vi "Run All Custom Tests.vi"(7 "Main VI":path, 8 "Error In":errorcluster, 9 "Grader Result in":T6, 10 "Challenge Config":T5, 11 "VIChallenge Config":T1={"AWS Credentials"={"AWSAccessKeyId"="", "Secret Key"=""}, "AWS Account Number"="", "SQS Jobs"=refnum, "SQS Status"=refnum, "Source Dir"=path "", "Working Dir"=path "", "Output Dir"=path "", "Archive Dir"=path "", "job"={"job_id"="", "challenge_id"="", "user_id"="", "s3_source_bucket"="", "s3_source_directory"="", "s3_source_filename"="", "status_queue_name"="", "username"=""}, "Database Ref"=refnum, "Challenge Dir"=path "", "Challenges"=[]}) -> (0 "Error Out":errorcluster, 1 "Grader Result":T6, 2 "Challenge Config":T5, 3 "VIChallenge Config":T1)   [LabVIEW 2013, in "VIChallenge.lvlib"]
doc: "This VI runs all custom tests for the given challenge and returns a single result."
uses:
  <vilib>/LabVIEW Hacker/VIChallenge/VIChallenge.lvlib
  <vilib>/LabVIEW Hacker/VIChallenge/Private/Grader/Type Defs/Grader Result.ctl
  <vilib>/LabVIEW Hacker/VIChallenge/Private/Type Defs/Database/Score.ctl
  <vilib>/LabVIEW Hacker/VIChallenge/Private/Grader/Type Defs/UTF Status.ctl
  <vilib>/LabVIEW Hacker/VIChallenge/Private/Grader/Type Defs/Challenge.ctl
  <vilib>/LabVIEW Hacker/VIChallenge/Private/Type Defs/VIChallenge Config.ctl
  <vilib>/National Instruments/NI Amazon Web Services (AWS) Toolkit for LabVIEW/SQS/VI Source/AWS SQS Class/AWS_SQS.lvclass
  <vilib>/National Instruments/NI Amazon Web Services (AWS) Toolkit for LabVIEW/AWS Core Lib/VI Source/Canonicals/AWS_Core Canonical Credentials/Canonical Credentials.lvclass
  <vilib>/National Instruments/NI Amazon Web Services (AWS) Toolkit for LabVIEW/AWS Core Lib/VI Source/Canonicals/AWS_Core Canonical Required Parameters/Canonical Required Parameters.lvclass
  <vilib>/National Instruments/NI Amazon Web Services (AWS) Toolkit for LabVIEW/SQS/VI Source/Canonicals/Canonical CreateQueue/Canonical CreateQueue.lvclass
  <vilib>/National Instruments/NI Amazon Web Services (AWS) Toolkit for LabVIEW/SQS/VI Source/Canonicals/Canonical ListQueues/Canonical ListQueues.lvclass
  <vilib>/National Instruments/NI Amazon Web Services (AWS) Toolkit for LabVIEW/SQS/VI Source/Canonicals/Canonical AddPermission/Canonical AddPermission.lvclass
  <vilib>/National Instruments/NI Amazon Web Services (AWS) Toolkit for LabVIEW/SQS/VI Source/Canonicals/Canonical ChangeMessageVisibility/Canonical ChangeMessageVisibility.lvclass
  <vilib>/National Instruments/NI Amazon Web Services (AWS) Toolkit for LabVIEW/SQS/VI Source/Canonicals/Canonical ChangeMessageVisibilityBatch/Canonical ChangeMessageVisibilityBatch.lvclass
  <vilib>/National Instruments/NI Amazon Web Services (AWS) Toolkit for LabVIEW/SQS/VI Source/Canonicals/Canonical DeleteMessage/Canonical DeleteMessage.lvclass
  <vilib>/National Instruments/NI Amazon Web Services (AWS) Toolkit for LabVIEW/SQS/VI Source/Canonicals/Canonical DeleteMessageBatch/Canonical DeleteMessageBatch.lvclass
  <vilib>/National Instruments/NI Amazon Web Services (AWS) Toolkit for LabVIEW/SQS/VI Source/Canonicals/Canonical GetQueueAttributes/Canonical GetQueueAttributes.lvclass
  <vilib>/National Instruments/NI Amazon Web Services (AWS) Toolkit for LabVIEW/SQS/VI Source/Canonicals/Canonical GetQueueUrl/Canonical GetQueueUrl.lvclass
  <vilib>/National Instruments/NI Amazon Web Services (AWS) Toolkit for LabVIEW/SQS/VI Source/Canonicals/Canonical ReceiveMessage/Canonical ReceiveMessage.lvclass
  <vilib>/National Instruments/NI Amazon Web Services (AWS) Toolkit for LabVIEW/SQS/VI Source/Canonicals/Canonical RemovePermission/Canonical RemovePermission.lvclass
  <vilib>/National Instruments/NI Amazon Web Services (AWS) Toolkit for LabVIEW/SQS/VI Source/Canonicals/Canonical SendMessage/Canonical SendMessage.lvclass
  <vilib>/National Instruments/NI Amazon Web Services (AWS) Toolkit for LabVIEW/SQS/VI Source/Canonicals/Canonical SendMessageBatch/Canonical SendMessageBatch.lvclass
  <vilib>/National Instruments/NI Amazon Web Services (AWS) Toolkit for LabVIEW/SQS/VI Source/Canonicals/Canonical SetQueueAttributes/Canonical SetQueueAttributes.lvclass
  <vilib>/National Instruments/NI Amazon Web Services (AWS) Toolkit for LabVIEW/AWS Core Lib/VI Source/Typedefs/AWS_AWS Credentials.ctl
  <vilib>/LabVIEW Hacker/VIChallenge/Private/Type Defs/JSON_job.ctl
  <vilib>/addons/database/Connection.llb/Conn ObjectReference.ctl
  <vilib>/National Instruments/NI Amazon Web Services (AWS) Toolkit for LabVIEW/AWS Core Lib/VI Source/AWS_Core.lvlib
  <vilib>/addons/database/NI_Database_API.lvlib
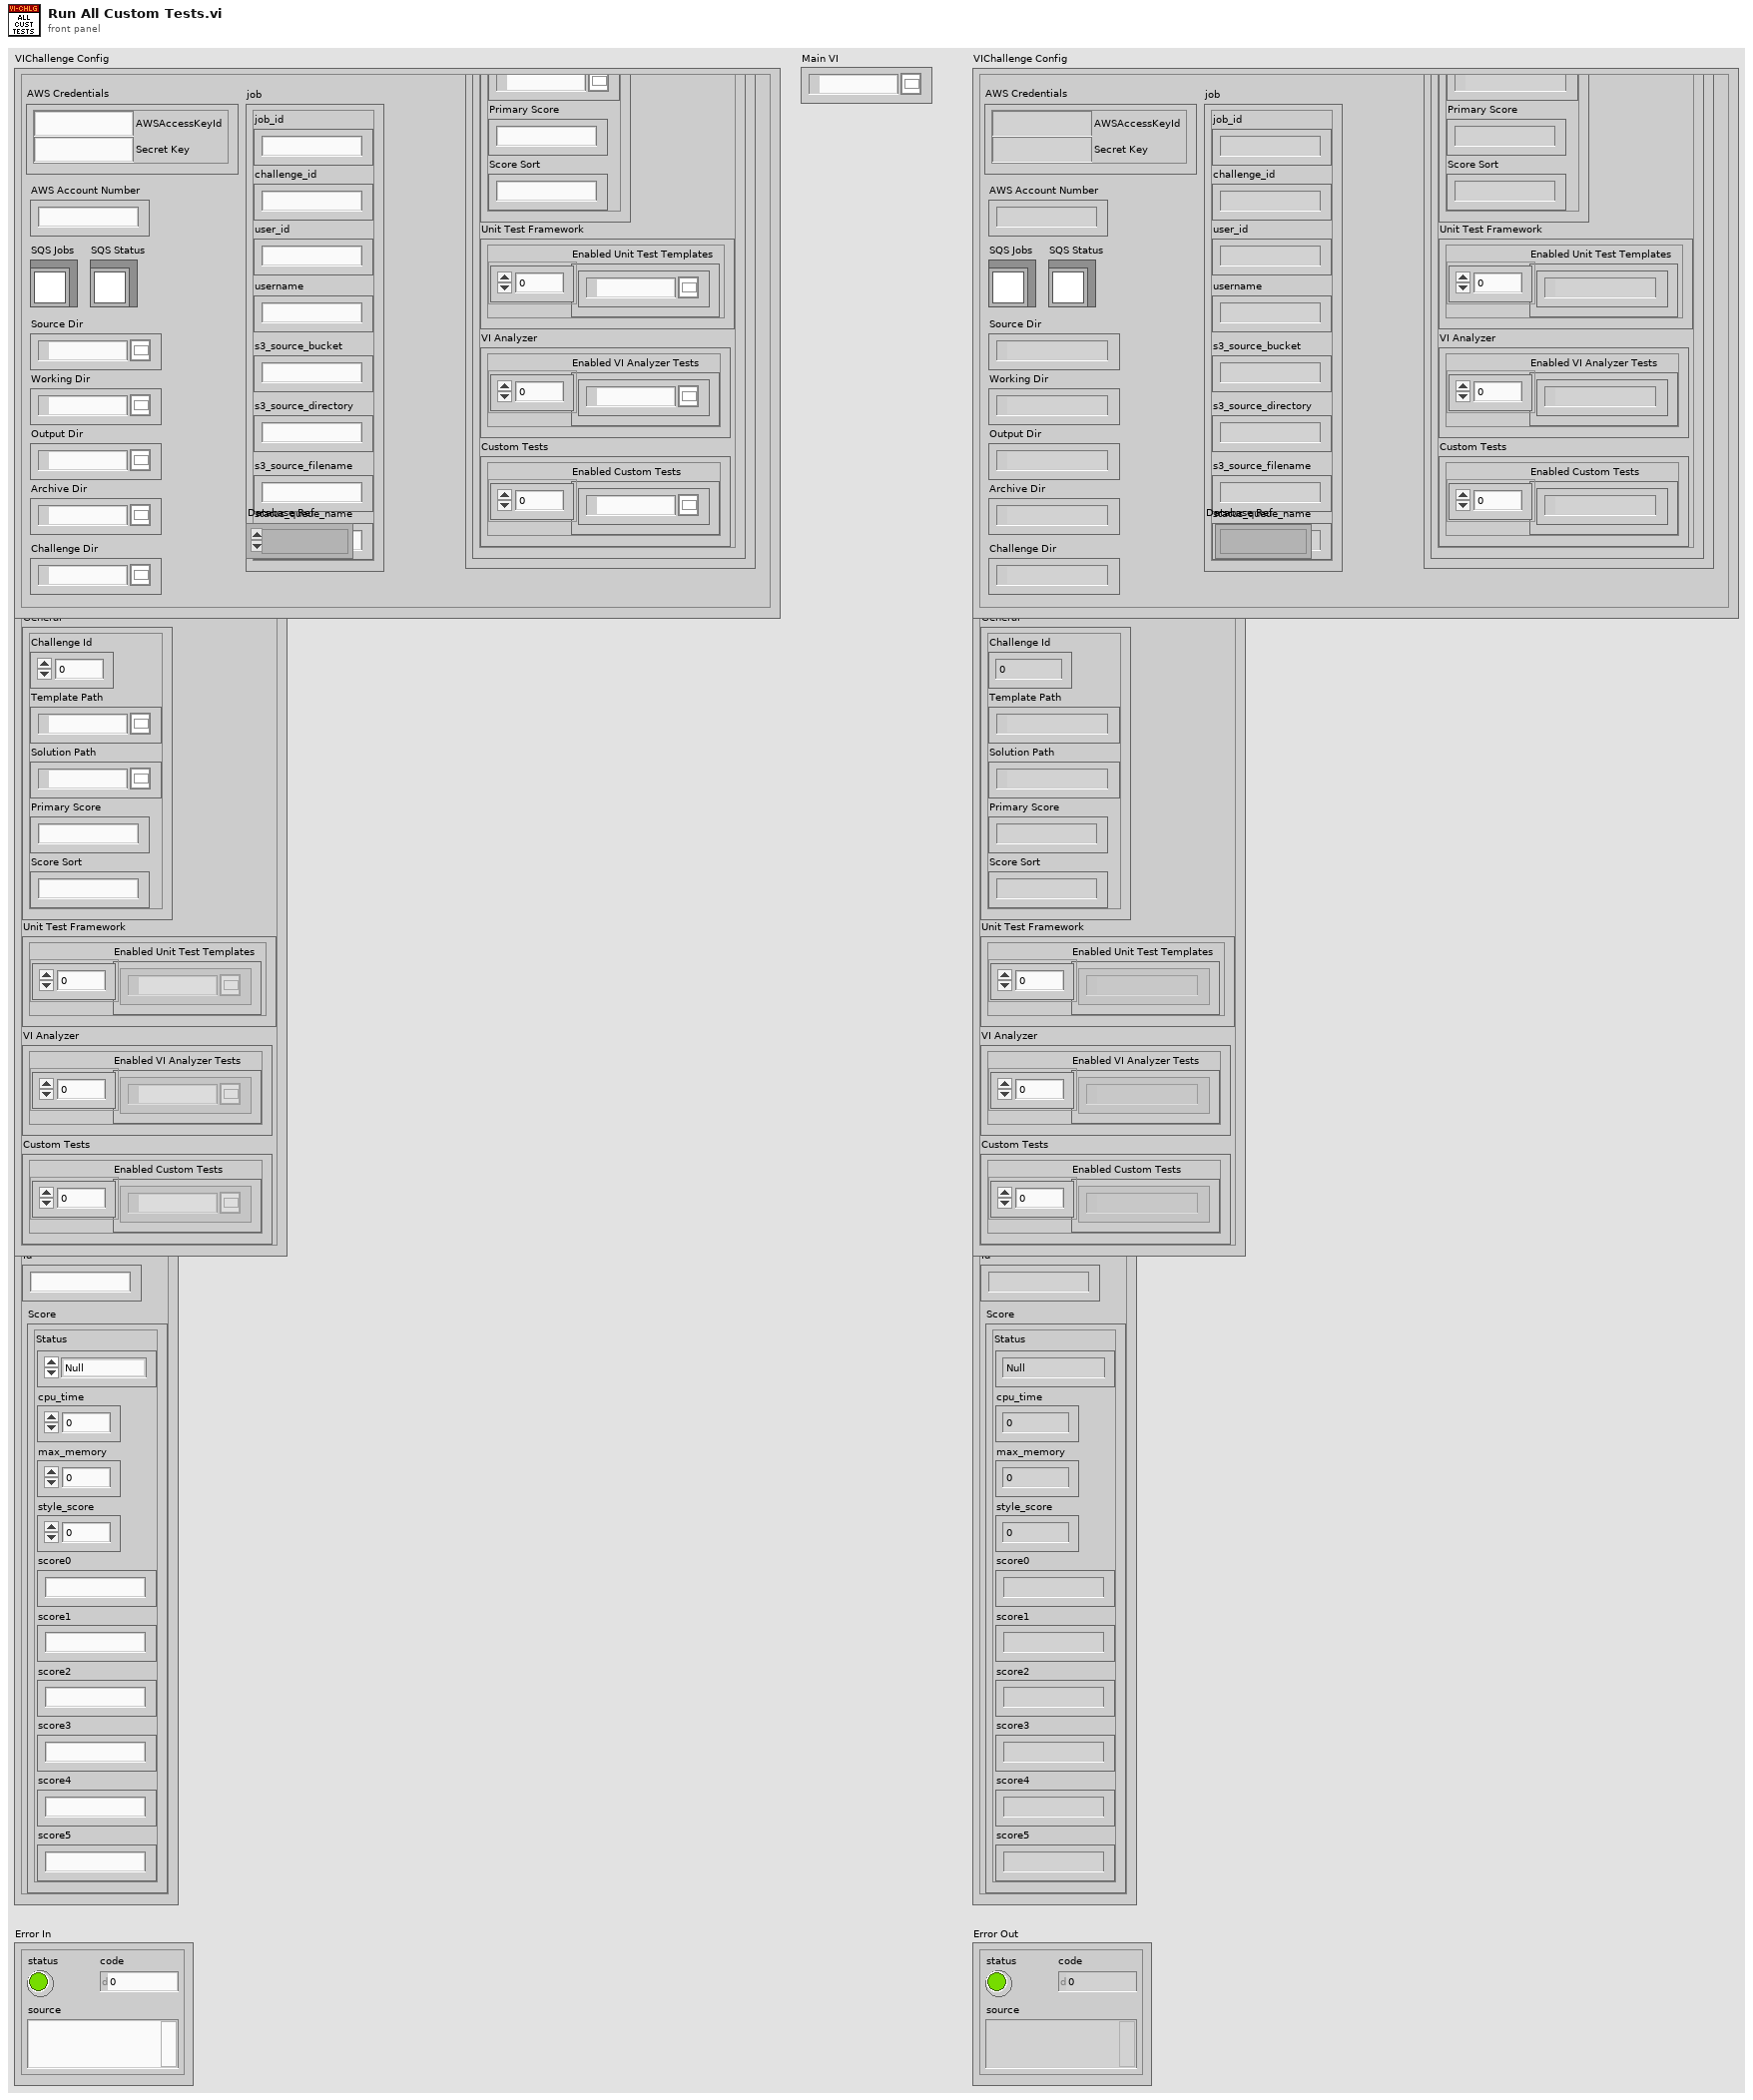
[diagram p1: front panel]
types:
  T1 = typedef "VIChallenge.lvlib/VIChallenge Config.ctl" = cluster{"AWS Credentials":T2, "AWS Account Number":string, "SQS Jobs":refnum<class "AWS_SQS.lvclass">, "SQS Status":refnum<class "AWS_SQS.lvclass">, "Source Dir":path, "Working Dir":path, "Output Dir":path, "Archive Dir":path, "job":T3, "Database Ref":T4, "Challenge Dir":path, "Challenges":T5[]}
  T2 = typedef "AWS_Core.lvlib/AWS_AWS Credentials.ctl" = cluster{"AWSAccessKeyId":string, "Secret Key":string}
  T3 = typedef "VIChallenge.lvlib/JSON_job.ctl" = cluster{"job_id":string, "challenge_id":string, "user_id":string, "s3_source_bucket":string, "s3_source_directory":string, "s3_source_filename":string, "status_queue_name":string, "username":string}
  T4 = typedef "NI_Database_API.lvlib/Conn ObjectReference.ctl" = refnum<k1>
  T5 = typedef "VIChallenge.lvlib/Challenge.ctl" = cluster{"General":cluster{"Challenge Id":i32, "Template Path":path, "Solution Path":path, "Primary Score":string, "Score Sort":string}, "Unit Test Framework":cluster{"Enabled Unit Test Templates":path[]}, "VI Analyzer":cluster{"Enabled VI Analyzer Tests":path[]}, "Custom Tests":cluster{"Enabled Custom Tests":path[]}}
  T6 = typedef "VIChallenge.lvlib/Grader Result.ctl" = cluster{"Id":string, "Score":T7}
  T7 = typedef "VIChallenge.lvlib/Score.ctl" = cluster{"Status":T8, "cpu_time":i32, "max_memory":i32, "style_score":i32, "score0":string, "score1":string, "score2":string, "score3":string, "score4":string, "score5":string}
  T8 = typedef "VIChallenge.lvlib/UTF Status.ctl" = enum16{"Null", "Passed", "Failed", "Error", "Skipped", "Not Processed"}
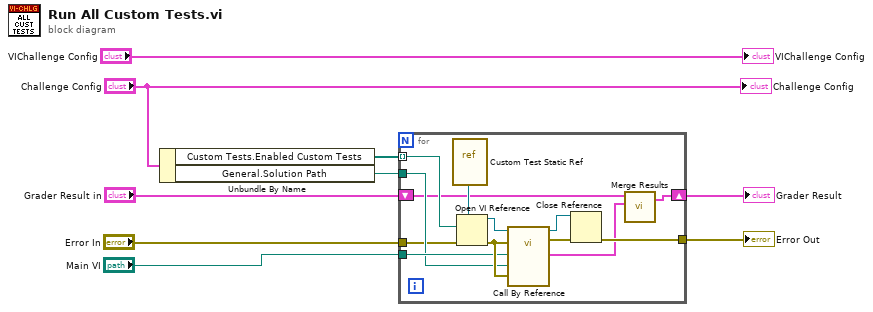
[diagram p0: block diagram]
diagram:
  n1 = Unbundle By Name("Challenge Config") -> ("Custom Tests.Enabled Custom Tests"=w3:path[], "General.Solution Path"=w4:path)
  n2 = for {
    tunnel: w3 -> [w21] mode=indexing
    tunnel: "Main VI" -> [w18]
    tunnel: w4 -> [w17]
    tunnel: [w14] -> w5
    tunnel: "Error In" -> [w13]
    shift-right: [w11] -> w7
    shift-left: "Grader Result in" -> [w12]
    n3 = vi-ref <vilib>:"Custom Test Static Ref.vi"() -> (w22:refnum<vi>)
    n4 = Open VI Reference(type specifier VI Refnum (for type only)=w22, vi path=w21, error in (no error)=w13) -> (vi reference=w20:refnum<vi>, error out=w19:errorcluster)  [unwired: 3 in]
    n5 = call-by-ref "?"(reference=w20, error in=w19, "Error In"=w19, "Solution VI"=w17, "User VI"=w18) -> (reference out=w15:refnum<vi>, error out=w16:errorcluster, "Results"=w10:T6)  [unwired: 1 in, 1 out]
    n6 = Close Reference(reference=w15, error in (no error)=w16) -> (error out=w14:errorcluster)
    n7 = call <vilib>:"Merge Results.vi"("Result 2"=w10, "Results 1"=w12) -> ("Results"=w11:T6)  [unwired: 3 in]
  }
  "Grader Result" <- w7
  "Error Out" <- w5
  "Challenge Config" <- "Challenge Config"
  "VIChallenge Config" <- "VIChallenge Config"
